vi "Load Digital Pattern Generation.vi"(6 "memory":refnum<k21>="Digital Pattern Gen Memory 0", 11 "load input.<user name>":T2) -> (0 "done":bool, 2 "load data":T1={"max address"=0.0, "memory"="Digital Pattern Gen Memory 0"})   [LabVIEW 2015, in "Engine Simulation Toolkit.lvlib" / "Digital Pattern Generation.lvlib"]
doc: "Loads data from NI VeriStand into the digital pattern generation memory. <b> This VI should be in an SCTL</b>\n\n<b>load input.<user name></b> - input for the component. NI VeriStand will set these values. create a control for this input. Replace <user name> with the name you wish this component to display as inside NI VeriStand. Make this name consistent for all controls, indicators, for all VIs of this component.\n<b>memory</b> - reference to a U16 memory of size 1024 or 2048. The memory holds edges, so half this value is the number of pulses the pattern can hold. The memory can be set to never arbitrate to save resources.\n\n<b>load data</b> - Information about the loaded memory that should be wired to Digital Pattern Generation.vi\n<b>done</b> - done loading signal. Wire this to the SCTL stop terminal."
uses:
  Digital Pattern Generation.lvlib
  Load Input.ctl
  Load Data.ctl
  <vilib>/rvi/Emulation/niFpgaSctlEmulationGetInTimedLoop.vi
  <vilib>/Utility/error.llb/Clear Errors.vi
  <vilib>/rvi/DataTransferAndStorage/Container/Common/niFpgaContainerExecOnDevCompGetState.vi
  <vilib>/rvi/Emulation/niFpgaEmulationIsFPGAContextNoSignature.vi
  <vilib>/rvi/DataTransferAndStorage/Container/Common/niFpgaContainerGetUniqueNameForEmu.vi
  <vilib>/rvi/Emulation/niFpgaProcessEmulError.vi
  <vilib>/rvi/errors/nirviReportUnexpectedCaseInternalError (U32).vi
  <vilib>/rvi/Memory/Memory_Emulation/niFpgaMemoryEmulationCacheClearOnFirstRun.vi
  <vilib>/rvi/Memory/Memory_Emulation/nirvimemoryEmulationManagerCache_MakeExclusive.vi
  <vilib>/rvi/Memory/Memory_Emulation/niFpgaMemoryEmulationValidateCache.vi
  <vilib>/rvi/Memory/Memory_Emulation/nirvimemoryEmulationManagerCache_InsertValue.vi
  <vilib>/rvi/Memory/Memory_Emulation/nirvimemoryEmulationManagerCache_ReleaseExclusive.vi
  <vilib>/rvi/Memory/Memory_Emulation/nirvimemoryEmulationManagerCache_GetValue.vi
  <vilib>/rvi/Memory/Memory_Emulation/nirvimemoryEmulationManagerCache_SetValue.vi
  <vilib>/rvi/Emulation/niFpgaSctlEmulationResourceMgr.vi
  <vilib>/rvi/DataTransferAndStorage/Container/XNode/niFpgaContainer.xnode
  <vilib>/rvi/Memory/Memory_Emulation/niFpgaMemoryEmulationRefIn.vi
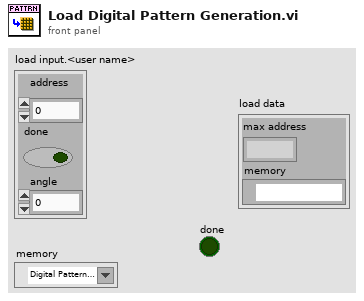
[diagram p1: front panel]
types:
  T1 = typedef "Engine Simulation Toolkit.lvlib/Digital Pattern Generation.lvlib/Load Data.ctl" = cluster{"max address":fxp<+,11,11>, "memory":refnum<k21>}
  T2 = typedef "Engine Simulation Toolkit.lvlib/Digital Pattern Generation.lvlib/Load Input.ctl" = cluster{"address":fxp<+,11,11>, "done":bool, "angle":u16}
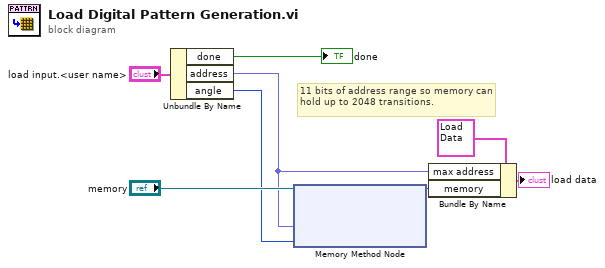
[diagram p0: block diagram]
diagram:
  # "11 bits of address range so memory can hold up to 2048 transitions."
  n1 = Unbundle By Name("load input.<user name>") -> ("done"=→"done":bool, "address"=w2:fxp<+,11,11>, "angle"=w1:u16)
  n2 = xnode ("Memory Method Node")("Address"=w2, "Data"=w1, "Memory In"="memory") -> ("Memory Out"=w3:refnum<k21>)
  n3 = Bundle By Name(cluster=T1 {"max address"=0.0, "memory"="Digital Pattern Gen Memory 0"} ("load data"), "max address"=w2, "memory"=w3) -> (→"load data":T1)
